vi "GF_ComputeLinearAverage.vi"(10 "Optional  ROI":dbl[](array[numeric]), 11 "Input Image":T1) -> (3 "Average Array":dbl[](array[numeric]))   [LabVIEW 2009]
uses:
  <vilib>/vision/Image Controls.llb/IMAQ Image.ctl
  <vilib>/Analysis/NI_AALBase.lvlib
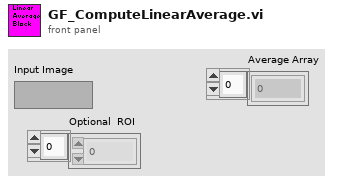
[diagram p1: front panel]
types:
  T1 = typedef "IMAQ Image.ctl" = refnum<image>
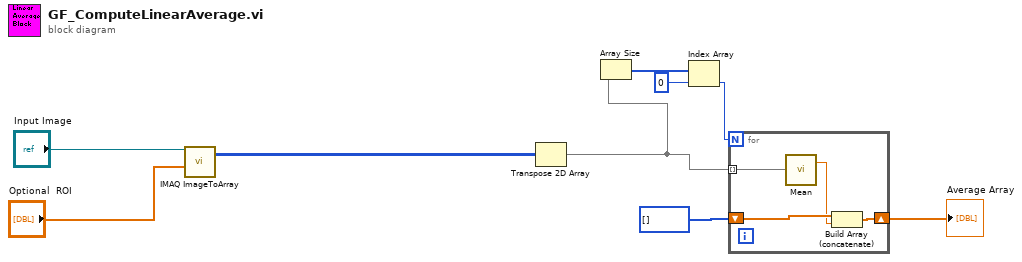
[diagram p0: block diagram]
diagram:
  n1 = call "IMAQ ImageToArray"("Optional Rectangle"="Optional  ROI", "Image"="Input Image") -> ("Image Pixels (I16)"=w2:i16[][])  [unwired: 2 in, 4 out]
  n2 = Transpose 2D Array(2D array=w2) -> (transposed array=w1:i16[][])
  n3 = Array Size(array=w1) -> (size(s)=w8:i32[])
  n4 = Index Array(array=w8, index=0) -> (element=w6:i32)
  n5 = for {
    N: w6 -> [_]
    tunnel: w1 -> [w10] mode=indexing
    shift-right: [w11] -> w5
    shift-left: i32[] [] -> [w13]
    n6 = call <vilib>:"Mean.vi"("X"=w10) -> ("mean"=w12:dbl)  [unwired: 1 out]
    n7 = Build Array (concatenate)(w13, w12) -> (w11:dbl[])
  }
  "Average Array" <- w5
